vi "ConfigurePacketWriter.vi"(2 "Filename":string caption="Filename (*.4pf)", 3 "NXT":T2={"Hardware"="NXT", "Flattened String"=""}, 7 "File Size":u32=2048 caption="File Size (2048)", 8 "Remote 1 Nodes":T1={"button 1"=TRUE, "button 2"=TRUE, "button 3"=TRUE, "button 4"=TRUE, "button 5"=TRUE, "button 6"=TRUE, "button 7"=TRUE, "button 8"=TRUE, "button 9"=TRUE, "button 10"=TRUE, "button 11"=TRUE, "button 12"=TRUE, "POV"=TRUE, "Left X"=TRUE, "Left Y"=TRUE, "Right X"=TRUE, "Right Y"=TRUE} caption="Remote 1 Nodes (All)", 9 "Remote 2 Nodes":T1={"button 1"=TRUE, "button 2"=TRUE, "button 3"=TRUE, "button 4"=TRUE, "button 5"=TRUE, "button 6"=TRUE, "button 7"=TRUE, "button 8"=TRUE, "button 9"=TRUE, "button 10"=TRUE, "button 11"=TRUE, "button 12"=TRUE, "POV"=TRUE, "Left X"=TRUE, "Left Y"=TRUE, "Right X"=TRUE, "Right Y"=TRUE} caption="Remote 2 Nodes (All)") -> (0 "NXT":T2={"Hardware"="NXT", "Flattened String"=""})   [LabVIEW 2010, in "Packet Recorder.lvlib"]
uses:
  Packet Recorder.lvlib
  <vilib>/NXT/Subs/LVHSConnector.ctl
  ConfigData.ctl
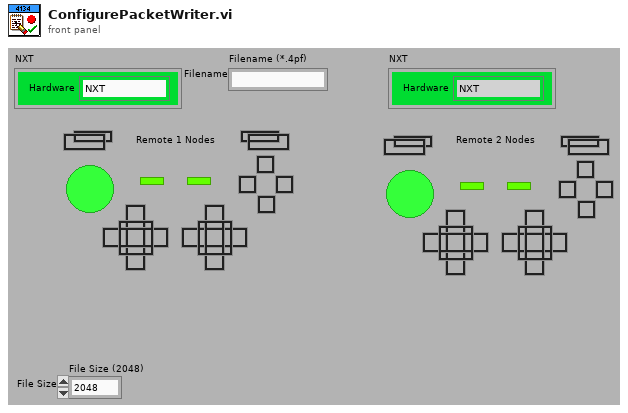
[diagram p1: front panel]
types:
  T1 = typedef "Packet Recorder.lvlib/ConfigData.ctl" = cluster{"button 1":bool, "button 2":bool, "button 3":bool, "button 4":bool, "button 5":bool, "button 6":bool, "button 7":bool, "button 8":bool, "button 9":bool, "button 10":bool, "button 11":bool, "button 12":bool, "POV":bool, "Left X":bool, "Left Y":bool, "Right X":bool, "Right Y":bool}
  T2 = typedef "LVHSConnector.ctl" = cluster{"Hardware":string, "Flattened String":string}
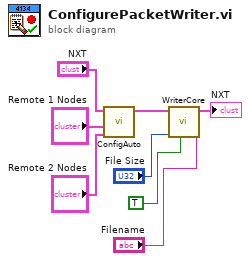
[diagram p0: block diagram]
diagram:
  n1 = call "ConfigAuto.vi"("Remote 2 Nodes"="Remote 2 Nodes", "Remote 1 Nodes"="Remote 1 Nodes", "NXT"="NXT") -> ("NXT"=w3:T2)  [unwired: 8 in]
  n2 = call "WriterCore.vi"("File Size"="File Size", "Initiational"=TRUE, "Filename"="Filename", "NXT"=w3) -> ("NXT"=→"NXT":T2)  [unwired: 7 in]
